vi "Software Cleanup.vi"(8 "error in (no error)":errorcluster) -> (0 "error out":errorcluster)   [LabVIEW 2013]
uses:
  <vilib>/Utility/error.llb/DialogType.ctl
  Peripherals Control/Shutter/Typedefs/Shutter state.ctl
  Typedefs/Save-Load enum.ctl
  Typedefs/Which path.ctl
  Global Variables/General Globals.vi
  Windows/Coordinates list window/Globals/Coord window-Globals.vi
  Configuration code/Calibration/Globals/gl_Calibration globals.vi
  Global Variables/gl_UI Ctrl Refs.vi
  Typedefs/Subpanel close request.ctl
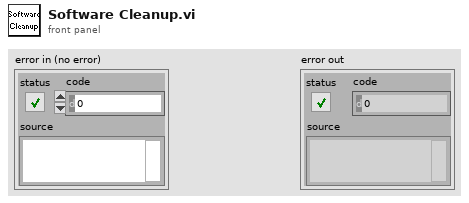
[diagram p1: front panel]
types:
  T1 = typedef "DialogType.ctl" = u16
  T2 = typedef "Which path.ctl" = enum16{"Configuration Files", "Calibration Files", "Images", "Setup.ini", "Loaded User profile.ini", "User's-Previous session.ini", "New user profile.ini", "Selected User profile.ini", "User profiles folder", "Power meter scaling.txt", "FOV Cal.ini"}
  T3 = typedef "Save-Load enum.ctl" = enum16{"Save to file", "Load from file", "Compare from file"}
  T4 = typedef "Shutter state.ctl" = enum16{"Closed/Disabled", "Open/Enabled"}
  T5 = typedef "Subpanel close request.ctl" = enum16{"Request subpanel close", "Just check subpanel is closed"}
  T6 = typedef "UI ctrl refs cluster.ctl" = cluster{"Top level VI path":path, "Top level VI ref":refnum<vi>, "User menu ref":refnum<k9>, "Sub Panel control":refnum<vi>, "Imaging Param Tab":refnum<vi>, "Occurrence-Start drivers":refnum<k4>, "Occurrence-Speed logging initialised":refnum<k4>, "Occurrence-XYZ stage initialised":refnum<k4>, "Exit button":refnum<vi>, "Status ind":refnum<vi>, "Return to Origin":refnum<vi>, "Speed Logging":refnum<vi>, "Time Lapse":refnum<vi>, "Live Imaging":refnum<vi>, "AOL Z Stack":refnum<vi>, "Motor Z Stack":refnum<vi>, "Funct Acq button":refnum<vi>, "Hard Shutter":refnum<vi>, "Virtual Shutter":refnum<vi>, "Laser Power":refnum<vi>, "AOL Mode":refnum<vi>, "Frame Size":refnum<vi>, "Field of View":refnum<vi>, "Dwell Time":refnum<vi>, "Zoom":refnum<vi>, "AOL Z":refnum<vi>, "Objective":refnum<vi>, "Axis":refnum<vi>, "Paths & Names":refnum<vi>, "Experiment folder path (ind.)":refnum<vi>, "Last State (Ind.)":refnum<vi>, "Laser wavelength ind (nm)":refnum<vi>, "Averages":refnum<vi>, "Angle (degrees)":refnum<vi>, "X centre":refnum<vi>, "Y centre":refnum<vi>, "Plane Mode":refnum<vi>, "# Planes":refnum<vi>, "Z Start":refnum<vi>, "Z Stop":refnum<vi>, "Z Step":refnum<vi>, "PMT 1":refnum<vi>, "PMT 2":refnum<vi>, "Stage XYZ Position":refnum<vi>, "Pockels@Z Start":refnum<vi>, "Pockels@Z Stop":refnum<vi>, "Obtain Z Start":refnum<vi>, "Obtain Z Stop":refnum<vi>, "Live stim.trig.period":refnum<vi>, "Live stim.trig.enable":refnum<vi>, "Funct. Acq. Pockels Modulation":refnum<vi>, "Enable Video Recording":refnum<vi>, "Video Record-Live Imaging":refnum<vi>, "Video Record-Funct acq":refnum<vi>, "AOL Z-stack Chirps Ready (ind)":refnum<vi>, "Center freq ind (nm)":refnum<vi>, "Logging queue (ind)":refnum<vi>, "Back aperture power (ind.)":refnum<vi>, "Power after objective (ind.)":refnum<vi>, "Switch user":refnum<vi>}
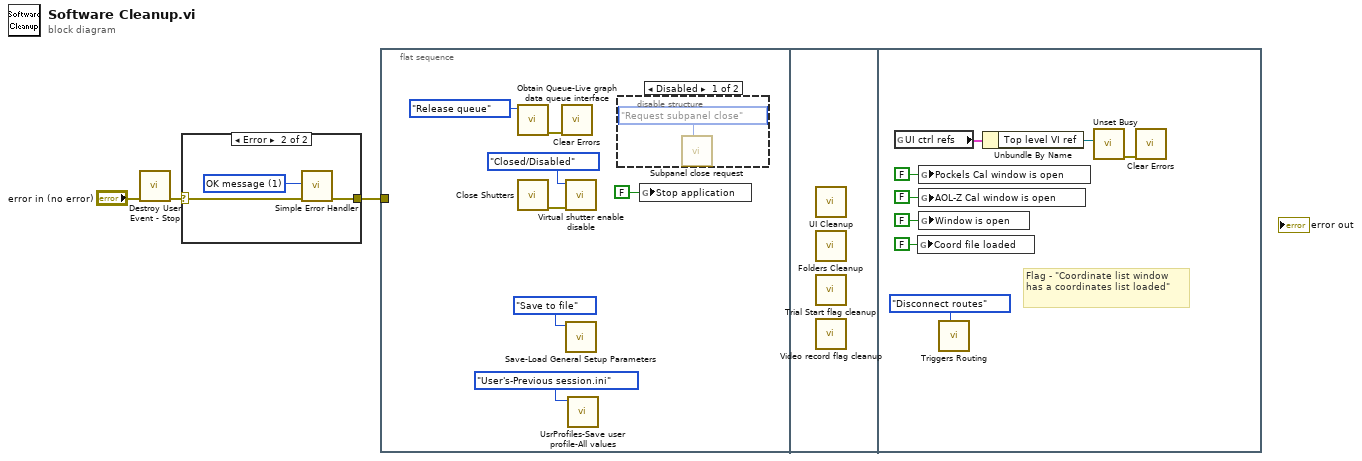
[diagram p0: block diagram]
diagram:
  n1 = call "Destroy User Event - Stop.vi"("Error In"="error in (no error)") -> ("Error Out"=w1:errorcluster)  [unwired: 10 in]
  n2 = case shown="Error" w1 {
    selector: w1 -> [w4 w5]
    tunnel: [w4 w7] -> w2
    frame No Error {
    }
    frame Error {
      w6 = T1 1 items=["no dialog", "OK message", "continue or stop message", "OK message + warnings", "continue/stop + warnings"] ("type of dialog (OK msg:1)")
      n3 = call <vilib>:"Simple Error Handler.vi"("type of dialog (OK msg:1)"=w6, "error in (no error)"=w5) -> ("error out"=w7:errorcluster)  [unwired: 3 in, 4 out]
    }
  }
  n4 = flat-sequence {
    tunnel: w2 -> [_]
    frame #0 {
      n5 = call "Obtain Queue-Live graph data queue interface.vi"("Function"=enum16{"None", "Release queue"}."Release queue") -> ("error out"=w13:errorcluster)  [unwired: 9 in, 1 out]
      n6 = call "Close Shutters.vi"() -> ("error out (no error)"=w10:errorcluster)  [unwired: 11 in]
      n7 = call <vilib>:"Clear Errors.vi"("error in (no error)"=w13) -> ()  [unwired: 6 in, 1 out]
      n8 = call "Virtual shutter enable disable.vi"("error in (no error)"=w10, "Virtual Shutter"=Shutter_state."Closed/Disabled") -> ()  [unwired: 9 in, 1 out]
      n9 = call "Save-Load General Setup Parameters.vi"("Function"=Save-Load_enum."Save to file") -> ()  [unwired: 10 in, 1 out]
      n10 = call "UsrProfiles-Save user profile-All values.vi"("Which file? (User profile.ini)"=Which_path."User's-Previous session.ini" ("Which file?")) -> ()  [unwired: 10 in, 1 out]
      n11 = disable-structure shown="Disabled" {
        frame Disabled {
          n12 = call "Subpanel close request.vi"("Function"=Subpanel_close_request."Request subpanel close") -> ()  [unwired: 10 in, 1 out]
        }
        frame Enabled {
        }
      }
      n13 = global write "General Globals.vi" "Stop application"(FALSE ("Stop application")) -> ()
    }
    frame #1 {
      n14 = call "UI Cleanup.vi"() -> ()  [unwired: 11 in, 1 out]
      n15 = call "Folders Cleanup.vi"() -> ()  [unwired: 11 in, 1 out]
      n16 = call "Trial Start flag cleanup.vi"() -> ()  [unwired: 12 in]
      n17 = call "Video record flag cleanup.vi"() -> ()  [unwired: 12 in]
    }
    frame #2 {
      # "Flag - \"Coordinate list window has a coordinates list loaded\""
      n18 = global read "gl_UI Ctrl Refs.vi" "UI ctrl refs"() -> (w22:T6)
      n19 = global write "Coord window-Globals.vi" "Coord file loaded"(FALSE ("Initialised")) -> ()
      n20 = global write "gl_Calibration globals.vi" "Pockels Cal window is open"(FALSE ("Motor Z calibr window is open")) -> ()
      n21 = global write "gl_Calibration globals.vi" "AOL-Z Cal window is open"(FALSE ("Motor Z calibr window is open")) -> ()
      n22 = global write "Coord window-Globals.vi" "Window is open"(FALSE ("Window is open")) -> ()
      n23 = call "Triggers Routing.vi"("Function"=enum16{"Connect routes", "Disconnect routes"}."Disconnect routes") -> ()  [unwired: 10 in, 1 out]
      n24 = Unbundle By Name(w22) -> ("Top level VI ref"=w21:refnum<vi>)
      n25 = call <vilib>:"Unset Busy.vi"("VI reference (current VI)"=w21) -> ("error out"=w23:errorcluster)  [unwired: 10 in]
      n26 = call <vilib>:"Clear Errors.vi"("error in (no error)"=w23) -> ()  [unwired: 6 in, 1 out]
    }
  }
